vi "Set VISA IO Session String.vi"(8 "error in (no error)":errorcluster, 9 "String":string="COM1", 10 "Variant in (type and name)":variant) -> (0 "error out":errorcluster, 2 "Variant":variant)   [LabVIEW 2011]
uses:
  JKI Reuse Candidates/Is an Error (error cluster)__JKI Error Handling.vi
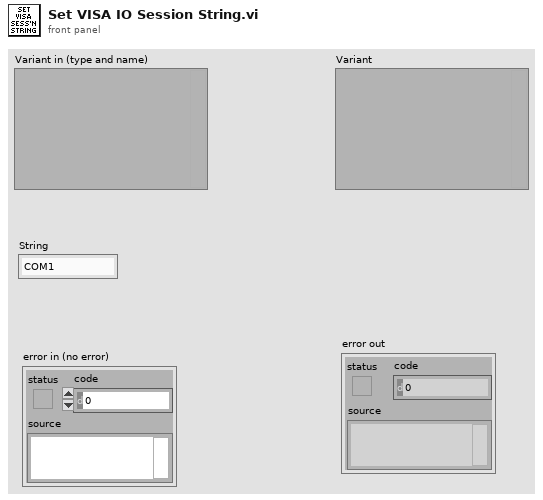
[diagram p1: front panel]
types:
  T1 = enum16{"Instr", "GPIB Instr", "VXI GPIB/VXI MBD Instr", "VXI GPIB/VXI/VME RBD Instr", "PXI Instr", "Serial Instr", "TCP/IP Instr", "USB Instr", "VXI/GPIB-VXI/VME MemAcc", "PXI MemAcc", "VXI/GPIB-VXI Backplane", "PXI Backplane", "VXI Servant", "GPIB BoardInterface", "GPIB Servant", "TCP/IP Socket", "USB Raw", "FireWire Instr"}
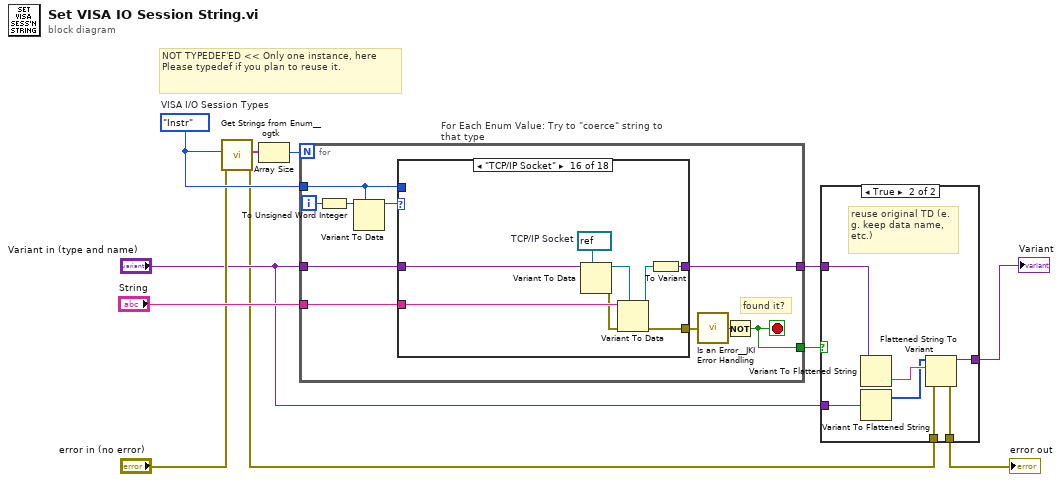
[diagram p0: block diagram]
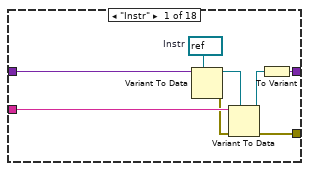
[diagram p3: hidden frame]
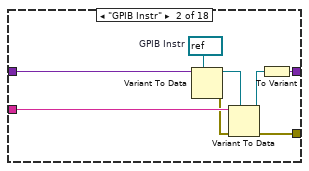
[diagram p4: hidden frame]
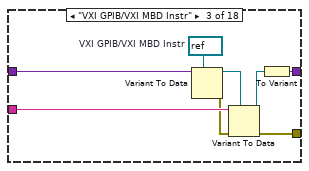
[diagram p5: hidden frame]
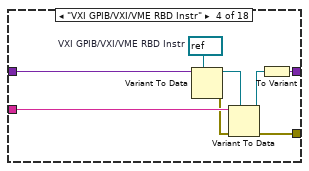
[diagram p6: hidden frame]
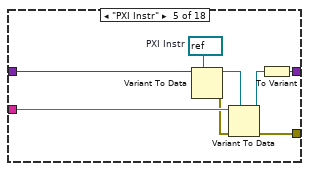
[diagram p7: hidden frame]
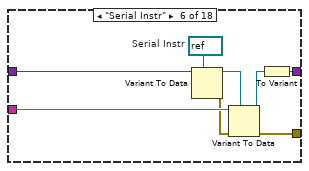
[diagram p8: hidden frame]
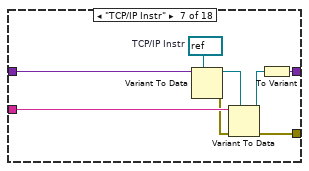
[diagram p9: hidden frame]
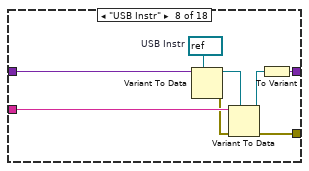
[diagram p10: hidden frame]
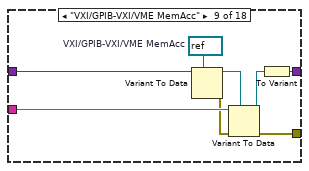
[diagram p11: hidden frame]
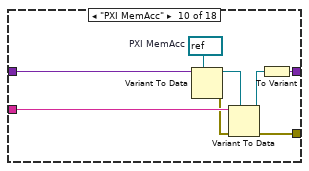
[diagram p12: hidden frame]
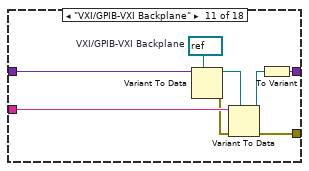
[diagram p13: hidden frame]
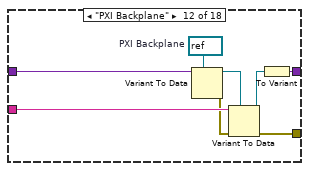
[diagram p14: hidden frame]
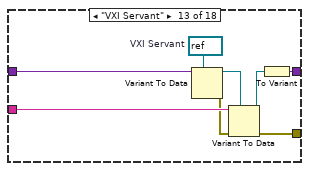
[diagram p15: hidden frame]
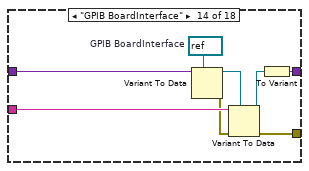
[diagram p16: hidden frame]
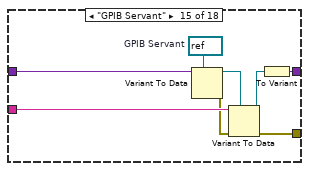
[diagram p17: hidden frame]
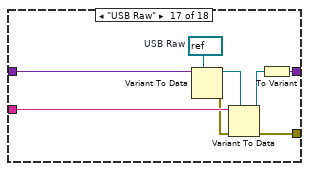
[diagram p18: hidden frame]
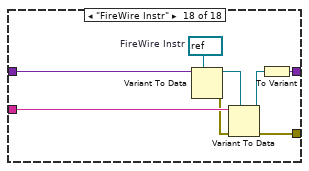
[diagram p19: hidden frame]
diagram:
  w9 = T1."Instr"  # VISA I/O Session Types
  # "NOT TYPEDEF'ED << Only one instance, here\nPlease typedef if you plan to reuse it."
  n1 = call <userlib>:"Get Strings from Enum__ogtk.vi"("error in (no error)"="error in (no error)", "Enum"=w9) -> ("error out"=w5:errorcluster, "Enum Strings"=w11:string[])  [unwired: 6 in, 2 out]
  n2 = Array Size(array=w11) -> (size(s)=w10:i32)
  n3 = for "For Each Enum Value: Try to \"coerce\" string to that type" {
    N: w10 -> [_]
    tunnel: w9 -> [w18]
    tunnel: "Variant in (type and name)" -> [w17]
    tunnel: [w14] -> w2
    tunnel: "String" -> [w13]
    tunnel: [w12] -> w1
    i -> [w21]
    stop <- w12 stop-if-true
    # "found it?"
    n4 = To Unsigned Word Integer(number=w21) -> (unsigned 16bit integer=w20:u16)
    n5 = Variant To Data(type=w18, Variant=w20) -> (data=w19:T1)  [unwired: 1 in, 1 out]
    n6 = case shown="\"TCP/IP Socket\"" w19 {
      tunnel: w18 -> [_ _ _ _ _ _ _ _ _ _ _ _ _ _ _ _ _ _]
      tunnel: w17 -> [w29 w37 w45 w53 w61 w69 w77 w85 w93 w101 w109 w117 w125 w133 w141 w149 w157 w165]
      tunnel: [w27 w35 w43 w51 w59 w67 w75 w83 w91 w99 w107 w115 w123 w131 w139 w147 w155 w163] -> w14
      tunnel: [w22 w30 w38 w46 w54 w62 w70 w78 w86 w94 w102 w110 w118 w126 w134 w142 w150 w158] -> w15
      tunnel: w13 -> [w24 w32 w40 w48 w56 w64 w72 w80 w88 w96 w104 w112 w120 w128 w136 w144 w152 w160]
      frame "Instr" {
        w28 = refnum<visa-resource-name> refnum  # Instr
        n7 = Variant To Data(type=w28, Variant=w29) -> (data=w26:refnum<visa-resource-name>, error out=w23:errorcluster)  [unwired: 1 in]
        n8 = Variant To Data(error in=w23, type=w26, Variant=w24) -> (data=w25:refnum<visa-resource-name>, error out=w22:errorcluster)
        n9 = To Variant(anything=w25) -> (Variant=w27:variant)
      }
      frame "GPIB Instr" {
        w36 = refnum<visa-resource-name> refnum  # GPIB Instr
        n10 = Variant To Data(type=w36, Variant=w37) -> (data=w34:refnum<visa-resource-name>, error out=w31:errorcluster)  [unwired: 1 in]
        n11 = Variant To Data(error in=w31, type=w34, Variant=w32) -> (data=w33:refnum<visa-resource-name>, error out=w30:errorcluster)
        n12 = To Variant(anything=w33) -> (Variant=w35:variant)
      }
      frame "VXI GPIB/VXI MBD Instr" {
        w44 = refnum<visa-resource-name> refnum  # VXI GPIB/VXI MBD Instr
        n13 = Variant To Data(type=w44, Variant=w45) -> (data=w42:refnum<visa-resource-name>, error out=w39:errorcluster)  [unwired: 1 in]
        n14 = Variant To Data(error in=w39, type=w42, Variant=w40) -> (data=w41:refnum<visa-resource-name>, error out=w38:errorcluster)
        n15 = To Variant(anything=w41) -> (Variant=w43:variant)
      }
      frame "VXI GPIB/VXI/VME RBD Instr" {
        w52 = refnum<visa-resource-name> refnum  # VXI GPIB/VXI/VME RBD Instr
        n16 = Variant To Data(type=w52, Variant=w53) -> (data=w50:refnum<visa-resource-name>, error out=w47:errorcluster)  [unwired: 1 in]
        n17 = Variant To Data(error in=w47, type=w50, Variant=w48) -> (data=w49:refnum<visa-resource-name>, error out=w46:errorcluster)
        n18 = To Variant(anything=w49) -> (Variant=w51:variant)
      }
      frame "PXI Instr" {
        w60 = refnum<visa-resource-name> refnum  # PXI Instr
        n19 = Variant To Data(type=w60, Variant=w61) -> (data=w58:refnum<visa-resource-name>, error out=w55:errorcluster)  [unwired: 1 in]
        n20 = Variant To Data(error in=w55, type=w58, Variant=w56) -> (data=w57:refnum<visa-resource-name>, error out=w54:errorcluster)
        n21 = To Variant(anything=w57) -> (Variant=w59:variant)
      }
      frame "Serial Instr" {
        w68 = refnum<visa-resource-name> refnum  # Serial Instr
        n22 = Variant To Data(type=w68, Variant=w69) -> (data=w66:refnum<visa-resource-name>, error out=w63:errorcluster)  [unwired: 1 in]
        n23 = Variant To Data(error in=w63, type=w66, Variant=w64) -> (data=w65:refnum<visa-resource-name>, error out=w62:errorcluster)
        n24 = To Variant(anything=w65) -> (Variant=w67:variant)
      }
      frame "TCP/IP Instr" {
        w76 = refnum<visa-resource-name> refnum  # TCP/IP Instr
        n25 = Variant To Data(type=w76, Variant=w77) -> (data=w74:refnum<visa-resource-name>, error out=w71:errorcluster)  [unwired: 1 in]
        n26 = Variant To Data(error in=w71, type=w74, Variant=w72) -> (data=w73:refnum<visa-resource-name>, error out=w70:errorcluster)
        n27 = To Variant(anything=w73) -> (Variant=w75:variant)
      }
      frame "USB Instr" {
        w84 = refnum<visa-resource-name> refnum  # USB Instr
        n28 = Variant To Data(type=w84, Variant=w85) -> (data=w82:refnum<visa-resource-name>, error out=w79:errorcluster)  [unwired: 1 in]
        n29 = Variant To Data(error in=w79, type=w82, Variant=w80) -> (data=w81:refnum<visa-resource-name>, error out=w78:errorcluster)
        n30 = To Variant(anything=w81) -> (Variant=w83:variant)
      }
      frame "VXI/GPIB-VXI/VME MemAcc" {
        w92 = refnum<visa-resource-name> refnum  # VXI/GPIB-VXI/VME MemAcc
        n31 = Variant To Data(type=w92, Variant=w93) -> (data=w90:refnum<visa-resource-name>, error out=w87:errorcluster)  [unwired: 1 in]
        n32 = Variant To Data(error in=w87, type=w90, Variant=w88) -> (data=w89:refnum<visa-resource-name>, error out=w86:errorcluster)
        n33 = To Variant(anything=w89) -> (Variant=w91:variant)
      }
      frame "PXI MemAcc" {
        w100 = refnum<visa-resource-name> refnum  # PXI MemAcc
        n34 = Variant To Data(type=w100, Variant=w101) -> (data=w98:refnum<visa-resource-name>, error out=w95:errorcluster)  [unwired: 1 in]
        n35 = Variant To Data(error in=w95, type=w98, Variant=w96) -> (data=w97:refnum<visa-resource-name>, error out=w94:errorcluster)
        n36 = To Variant(anything=w97) -> (Variant=w99:variant)
      }
      frame "VXI/GPIB-VXI Backplane" {
        w108 = refnum<visa-resource-name> refnum  # VXI/GPIB-VXI Backplane
        n37 = Variant To Data(type=w108, Variant=w109) -> (data=w106:refnum<visa-resource-name>, error out=w103:errorcluster)  [unwired: 1 in]
        n38 = Variant To Data(error in=w103, type=w106, Variant=w104) -> (data=w105:refnum<visa-resource-name>, error out=w102:errorcluster)
        n39 = To Variant(anything=w105) -> (Variant=w107:variant)
      }
      frame "PXI Backplane" {
        w116 = refnum<visa-resource-name> refnum  # PXI Backplane
        n40 = Variant To Data(type=w116, Variant=w117) -> (data=w114:refnum<visa-resource-name>, error out=w111:errorcluster)  [unwired: 1 in]
        n41 = Variant To Data(error in=w111, type=w114, Variant=w112) -> (data=w113:refnum<visa-resource-name>, error out=w110:errorcluster)
        n42 = To Variant(anything=w113) -> (Variant=w115:variant)
      }
      frame "VXI Servant" {
        w124 = refnum<visa-resource-name> refnum  # VXI Servant
        n43 = Variant To Data(type=w124, Variant=w125) -> (data=w122:refnum<visa-resource-name>, error out=w119:errorcluster)  [unwired: 1 in]
        n44 = Variant To Data(error in=w119, type=w122, Variant=w120) -> (data=w121:refnum<visa-resource-name>, error out=w118:errorcluster)
        n45 = To Variant(anything=w121) -> (Variant=w123:variant)
      }
      frame "GPIB BoardInterface" {
        w132 = refnum<visa-resource-name> refnum  # GPIB BoardInterface
        n46 = Variant To Data(type=w132, Variant=w133) -> (data=w130:refnum<visa-resource-name>, error out=w127:errorcluster)  [unwired: 1 in]
        n47 = Variant To Data(error in=w127, type=w130, Variant=w128) -> (data=w129:refnum<visa-resource-name>, error out=w126:errorcluster)
        n48 = To Variant(anything=w129) -> (Variant=w131:variant)
      }
      frame "GPIB Servant" {
        w140 = refnum<visa-resource-name> refnum  # GPIB Servant
        n49 = Variant To Data(type=w140, Variant=w141) -> (data=w138:refnum<visa-resource-name>, error out=w135:errorcluster)  [unwired: 1 in]
        n50 = Variant To Data(error in=w135, type=w138, Variant=w136) -> (data=w137:refnum<visa-resource-name>, error out=w134:errorcluster)
        n51 = To Variant(anything=w137) -> (Variant=w139:variant)
      }
      frame "TCP/IP Socket" {
        w148 = refnum<visa-resource-name> refnum  # TCP/IP Socket
        n52 = Variant To Data(type=w148, Variant=w149) -> (data=w146:refnum<visa-resource-name>, error out=w143:errorcluster)  [unwired: 1 in]
        n53 = Variant To Data(error in=w143, type=w146, Variant=w144) -> (data=w145:refnum<visa-resource-name>, error out=w142:errorcluster)
        n54 = To Variant(anything=w145) -> (Variant=w147:variant)
      }
      frame "USB Raw" {
        w156 = refnum<visa-resource-name> refnum  # USB Raw
        n55 = Variant To Data(type=w156, Variant=w157) -> (data=w154:refnum<visa-resource-name>, error out=w151:errorcluster)  [unwired: 1 in]
        n56 = Variant To Data(error in=w151, type=w154, Variant=w152) -> (data=w153:refnum<visa-resource-name>, error out=w150:errorcluster)
        n57 = To Variant(anything=w153) -> (Variant=w155:variant)
      }
      frame "FireWire Instr" {
        w164 = refnum<visa-resource-name> refnum  # FireWire Instr
        n58 = Variant To Data(type=w164, Variant=w165) -> (data=w162:refnum<visa-resource-name>, error out=w159:errorcluster)  [unwired: 1 in]
        n59 = Variant To Data(error in=w159, type=w162, Variant=w160) -> (data=w161:refnum<visa-resource-name>, error out=w158:errorcluster)
        n60 = To Variant(anything=w161) -> (Variant=w163:variant)
      }
    }
    n61 = call-poly "Is an Error__JKI Error Handling.vi"("error in"=w15) -> ("error?"=w16:bool)  [unwired: 8 in]
    n62 = Not(x=w16) -> (.not. x?=w12:bool)
  }
  n63 = case shown="True" w1 {
    tunnel: "Variant in (type and name)" -> [w166 w174]
    tunnel: w5 -> [w167 w171]
    tunnel: [w167 w170] -> w4
    tunnel: [w166 w169] -> w3
    tunnel: w2 -> [_ w168]
    frame False {
      # "Pass out original"
    }
    frame True {
      # "reuse original TD (e.g. keep data name, etc.)"
      n64 = Variant To Flattened String(Variant=w168) -> (data string=w173:string)  [unwired: 1 out]
      n65 = Variant To Flattened String(Variant=w174) -> (1:w172:i16[])  [unwired: 1 out]
      n66 = Flattened String To Variant(4:w171, 6:w173, 7:w172) -> (0:w170:errorcluster, 3:w169:variant)
    }
  }
  "Variant" <- w3
  "error out" <- w4
